vi "GetBoxTemps.vi"(3 "error in (no error)":errorcluster) -> (0 "error out":errorcluster, 1 "Outside Box":dbl format="%#.10f", 2 "InsideBox":dbl format="%#.10f", 4 "String_Temp_NoiseBoxes":string)   [LabVIEW 2009]
doc: "Read multiple box temperatures."
panel:
  in  "SCPI command":string="sens:volt:dc:nplc 10,(@1019:1020)\nconf:volt:dc 10,0.0001,(@1019:1020)\nrout:scan (@1019:1020)\ninit\n"
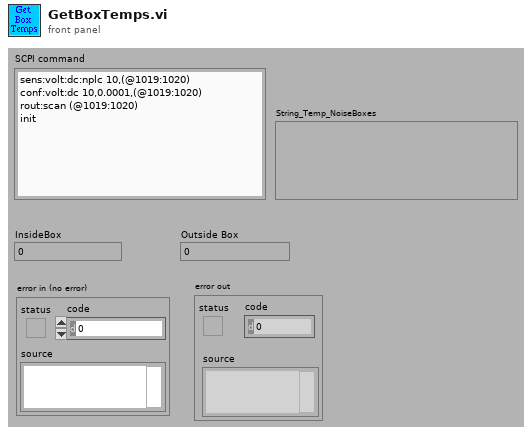
[diagram p1: front panel]
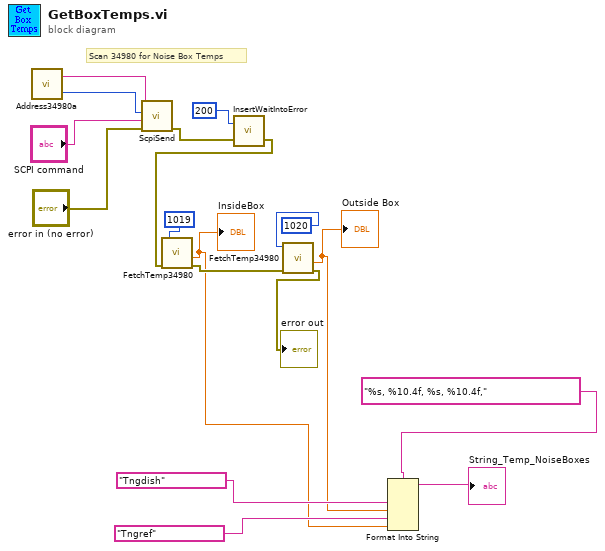
[diagram p0: block diagram]
diagram:
  # "Scan 34980 for Noise Box Temps"
  n1 = call "Address34980a.vi"() -> ("Port"=w14:i32, "IP address"=w15:string)  [unwired: 2 in]
  n2 = call "ScpiSend.vi"("error in (no error)"="error in (no error)", "Command"="SCPI command", "TCP port"=w14, "IP Address"=w15) -> ("error out"=w11:errorcluster)  [unwired: 7 in]
  n3 = call "InsertWaitIntoError.vi"("error in (no error)"=w11, "Wait (msecs)"=200) -> ("error out"=w10:errorcluster)  [unwired: 1 in]
  n4 = call "FetchTemp34980.vi"("error in (no error)"=w10, "Circuit ID"=1019) -> ("Error out"=w8:errorcluster, "Temp C"=w2:dbl)  [unwired: 2 in, 2 out]
  "InsideBox" <- w2
  n5 = call "FetchTemp34980.vi"("error in (no error)"=w8, "Circuit ID"=1020) -> ("Error out"=→"error out":errorcluster, "Temp C"=w3:dbl)  [unwired: 2 in, 2 out]
  "Outside Box" <- w3
  n6 = Format Into String(format string="%s, %10.4f, %s, %10.4f,", "Tngdish", w3, "Tngref", w2) -> (resulting string=→"String_Temp_NoiseBoxes":string)  [unwired: 2 in, 1 out]
